vi "FPGA_AIWriteConfig.vi"(8 "error in (no error)":errorcluster, 9 "Scan Size":u8, 10 "Convert Rate":u32, 11 "AI Reference":T1) -> (0 "error out":errorcluster, 3 "AI Reference":T1)   [LabVIEW 2017]
uses:
  <vilib>/Rock Robotics/SystemInterfaces/AI/FPGA_AIDevRef.ctl
  <vilib>/Rock Robotics/SystemInterfaces/System/FPGA_SystemFPGA Ref Global.vi
  <vilib>/Utility/error.llb/Error Cluster From Error Code.vi
  <vilib>/rvi/errors/niLvFpgaAdjustHostInterfaceError.vi
  <vilib>/rvi/interface/nirviReadWriteControl/nirviReadWriteControl.xnode
  <vilib>/Rock Robotics/SystemInterfaces/System/FPGA_SystemFRC FPGA Ref.ctl
  <vilib>/rvi/interface/Simulation/niFpgaSimulationCallBeginRW.vi
  NiFpgaLv.dll
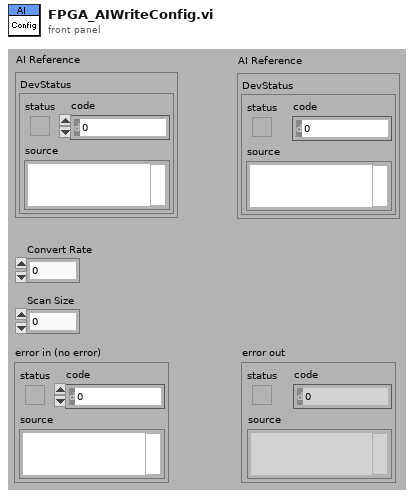
[diagram p1: front panel]
types:
  T1 = typedef "FPGA_AIDevRef.ctl" = cluster{"DevStatus":errorcluster}
  T2 = typedef "FPGA_SystemFRC FPGA Ref.ctl" = refnum<k20>
  T3 = cluster{"ScanSize":fxp<+,3,3>, "ConvertRate":fxp<+,26,26>}
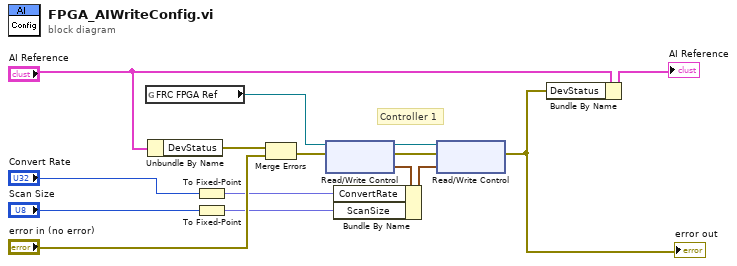
[diagram p0: block diagram]
diagram:
  # "Controller 1"
  n1 = global read "FPGA_SystemFPGA Ref Global.vi" "FRC FPGA Ref"() -> (w2:T2)
  n2 = Unbundle By Name("AI Reference") -> ("DevStatus"=w8:errorcluster)
  n3 = To Fixed-Point(number="Convert Rate") -> (fixed-point=w10:fxp<+,26,26>)  [unwired: 1 out]
  n4 = To Fixed-Point(number="Scan Size") -> (fixed-point=w9:fxp<+,3,3>)  [unwired: 1 out]
  n5 = Merge Errors(w8, "error in (no error)") -> (w7:errorcluster)
  n6 = xnode "Read/Write Control"("FPGA VI Reference In"=w2, "error in"=w7) -> ("FPGA VI Reference Out"=w5:T2, "error out"=w6:errorcluster, "AI.Config"=w4:T3)
  n7 = Bundle By Name(cluster=w4, "ConvertRate"=w10, "ScanSize"=w9) -> (w3:T3)
  n8 = xnode "Read/Write Control"("FPGA VI Reference In"=w5, "error in"=w6, "AI.Config"=w3) -> ("error out"=w14:errorcluster)  [unwired: 1 out]
  "error out" <- w14
  n9 = Bundle By Name(cluster="AI Reference", "DevStatus"=w14) -> (→"AI Reference":T1)
